vi "Flow Tags.vi"(11 "Flow Module Configs":T1[](array[typedef]) {"Settings"."Bronkhorst M14 Settings"."Smoothing Steps" min=1 step=1; "Settings"."Bronkhorst M13 Settings"."Smoothing Steps" min=1 step=1}) -> (1 "Flow Tags":T6, 2 "Flow Module Tags Array":T6[](array[typedef]), 3 "All  Numeric Tags 4":string[](array[string]), 4 "All Boolean Tags 4":string[](array[string]))   [LabVIEW 2018]
uses:
  Bronkhorst M14 Flow Meter/Tag Cluster.ctl
  Flow Module Folder/Feed Module/Controls/Flow Module Config Cluster.ctl
  <vilib>/Utility/miscctls.llb/LVPoint32TypeDef.ctl
  Flow Module Folder/Feed Module/Controls/Flow Module Settings Cluster.ctl
  Bronkhorst M13 Flow Meter/Settings Cluster.ctl
  Bronkhorst M14 Flow Meter/Settings Cluster.ctl
  Flow Module Folder/Flow Module.lvlib
  Bronkhorst M13 Flow Meter/Bronkhorst M13 Flow Meter.lvlib
  Bronkhorst M14 Flow Meter/Bronkhorst M14 Flow Meter.lvlib
panel:
  # "Flow Meter Settings"
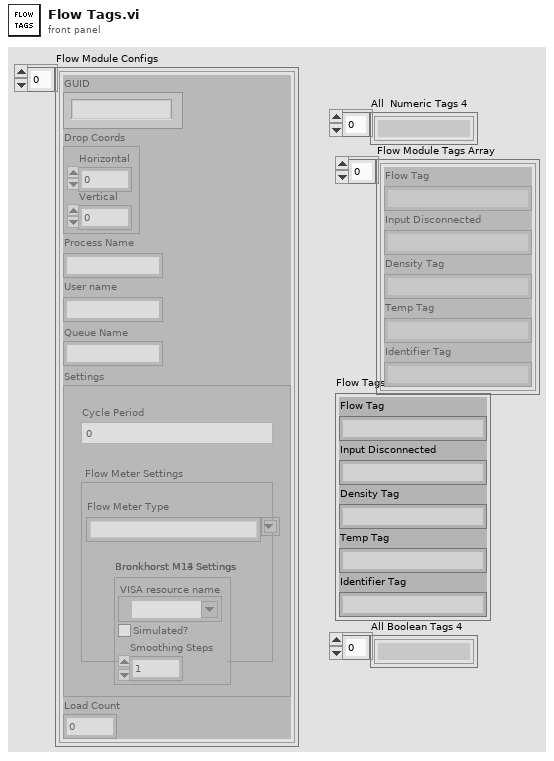
[diagram p1: front panel]
types:
  T1 = typedef "Flow Module.lvlib/Flow Module Config Cluster.ctl" = cluster{"GUID":string, "Drop Coords":T2, "Process Name":string, "User name":string, "Queue Name":string, "Settings":T3, "Load Count":i32}
  T2 = typedef "LVPoint32TypeDef.ctl" = cluster{"Horizontal":i32, "Vertical":i32}
  T3 = typedef "Flow Module.lvlib/Flow Module Settings Cluster.ctl" = cluster{"Cycle Period":dbl, "Flow Meter Type":string, "Bronkhorst M13 Settings":T4, "Bronkhorst M14 Settings":T5}
  T4 = typedef "Bronkhorst M13 Flow Meter.lvlib/Settings Cluster.ctl" = cluster{"VISA resource name":refnum<visa-resource-name>, "Simulated?":bool, "Smoothing Steps":i32}
  T5 = typedef "Bronkhorst M14 Flow Meter.lvlib/Settings Cluster.ctl" = cluster{"VISA resource name":refnum<visa-resource-name>, "Simulated?":bool, "Smoothing Steps":i32}
  T6 = typedef "Flow Module.lvlib/Tag Cluster.ctl" = cluster{"Flow Tag":string, "Input Disconnected":string, "Density Tag":string, "Temp Tag":string, "Identifier Tag":string}
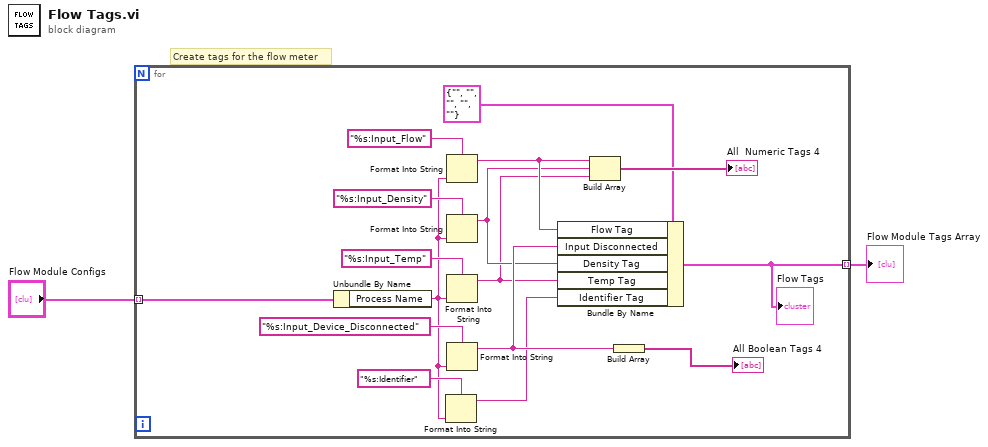
[diagram p0: block diagram]
diagram:
  # "Create tags for the flow meter"
  n1 = for {
    tunnel: "Flow Module Configs" -> [w7] mode=indexing
    tunnel: [w6] -> w2 mode=indexing
    n2 = Unbundle By Name(w7) -> ("Process Name"=w4:string)
    n3 = Format Into String(format string="%s:Identifier", w4) -> (resulting string=w3:string)  [unwired: 2 in, 1 out]
    n4 = Format Into String(format string="%s:Input_Flow", w4) -> (resulting string=w14:string)  [unwired: 2 in, 1 out]
    n5 = Format Into String(format string="%s:Input_Density", w4) -> (resulting string=w11:string)  [unwired: 2 in, 1 out]
    n6 = Format Into String(format string="%s:Input_Temp", w4) -> (resulting string=w8:string)  [unwired: 2 in, 1 out]
    n7 = Format Into String(format string="%s:Input_Device_Disconnected", w4) -> (resulting string=w13:string)  [unwired: 2 in, 1 out]
    n8 = Bundle By Name(cluster=T6 {"Flow Tag"="", "Input Disconnected"="", "Density Tag"="", "Temp Tag"="", "Identifier Tag"=""} ("Flow Tags 2"), "Flow Tag"=w14, "Input Disconnected"=w13, "Density Tag"=w11, "Temp Tag"=w8, "Identifier Tag"=w3) -> (w6:T6)
    "Flow Tags" <- w6
    n9 = Build Array(w14, w11, w8) -> (→"All  Numeric Tags 4":string[])
    n10 = Build Array(w13) -> (→"All Boolean Tags 4":string[])
  }
  "Flow Module Tags Array" <- w2
